vi "Create Schedule File (Main).vi"(0 "Team Info":T2, 5 "# of Fields":i32=1 min=1, 9 "Matches Per Team":i32=1 min=1, 11 "Back To Back Interval":i32 min=0) -> (4 "Match Array (indices)":i32[][](array[numeric]), 6 "# of Teams":i32, 8 "Team Info Out":T2, 10 "# of Quadrants":i32, 14 "Max H2H":i32, 15 "Total # of Matches":i32)   [LabVIEW 2013]
uses:
  Team Data Array.ctl
panel:
  in  "Tab Control":T1(tab)
  in  "Create schedule.csv":bool
  in  "Create By-Match CSV":bool
  in  "Cancel Button":bool
  in  "Create By-team CSV":bool
  out "error out":errorcluster
  in  "error in (no error)":errorcluster
  out "Progress":dbl(slide) scale=0.0..1.0
  in  "Output Folder":path
  in  "Entry Method":enum16{"Team Data Array", "Schedule Path"}(ring)
  in  "Team Info / Schedule File":path=path "Z:/Code/LabVIEW/[GEN2] FLL/schedule.csv"
  out "Flag Array":bool[][](array[boolean])
  out "H2H Flag":bool[][](array[boolean])
  out "H2H":i32[][](array[numeric])
  out "Match Array (numbers)":i32[][](array[numeric])
  out "By-Match Table":string[][](table)
  out "By-Team Table":string[][](table)
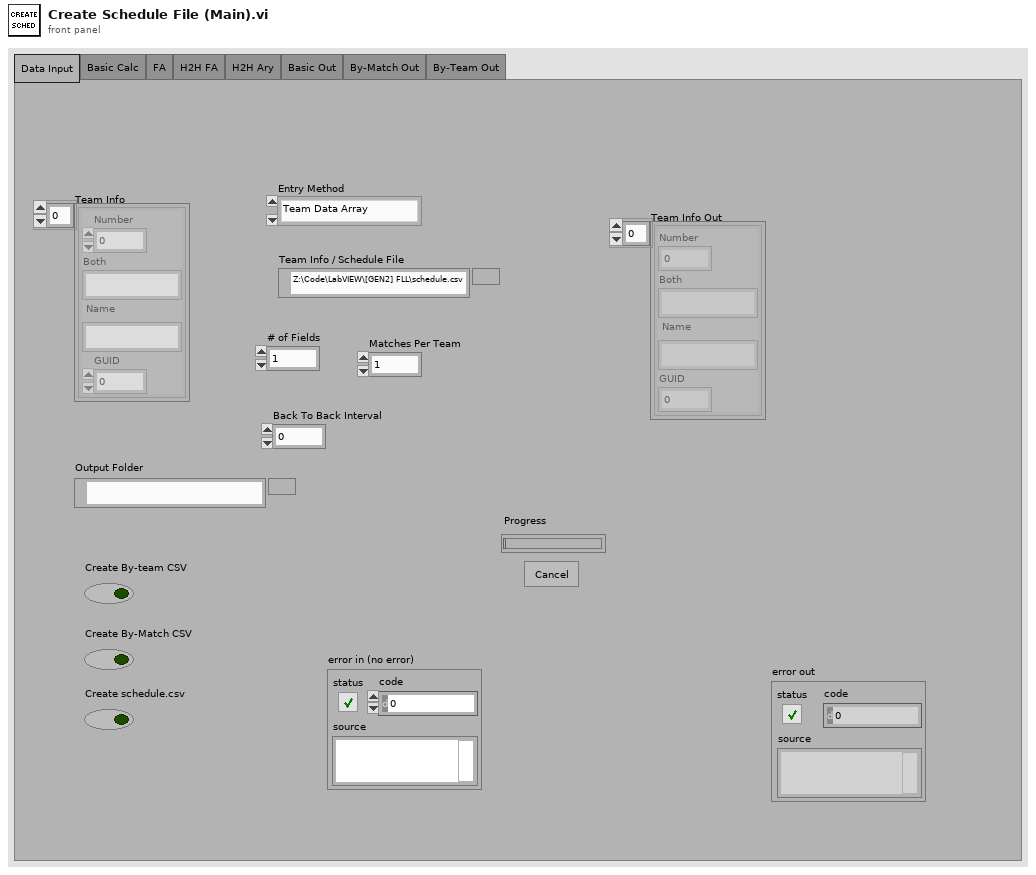
[diagram p1: front panel]
types:
  T1 = enum32{"Data Input", "Basic Calc", "FA", "H2H FA", "H2H Ary", "Basic Out", "By-Match Out", "By-Team Out"}
  T2 = typedef "Team Data Array.ctl" = cluster{"Number":u16, "Both":string, "Name":string, "GUID":u16}[]
  T3 = cluster{"Number":u16, "Both":string, "Name":string, "GUID":u16}
  T4 = cluster{"Total # of Matches":i32, "# of Fields":i32, "Matches Per Team":i32, "# of Teams":i32}
  T5 = cluster{"Row Headers":string[], "Column Headers":string[], "Items":string[][]}
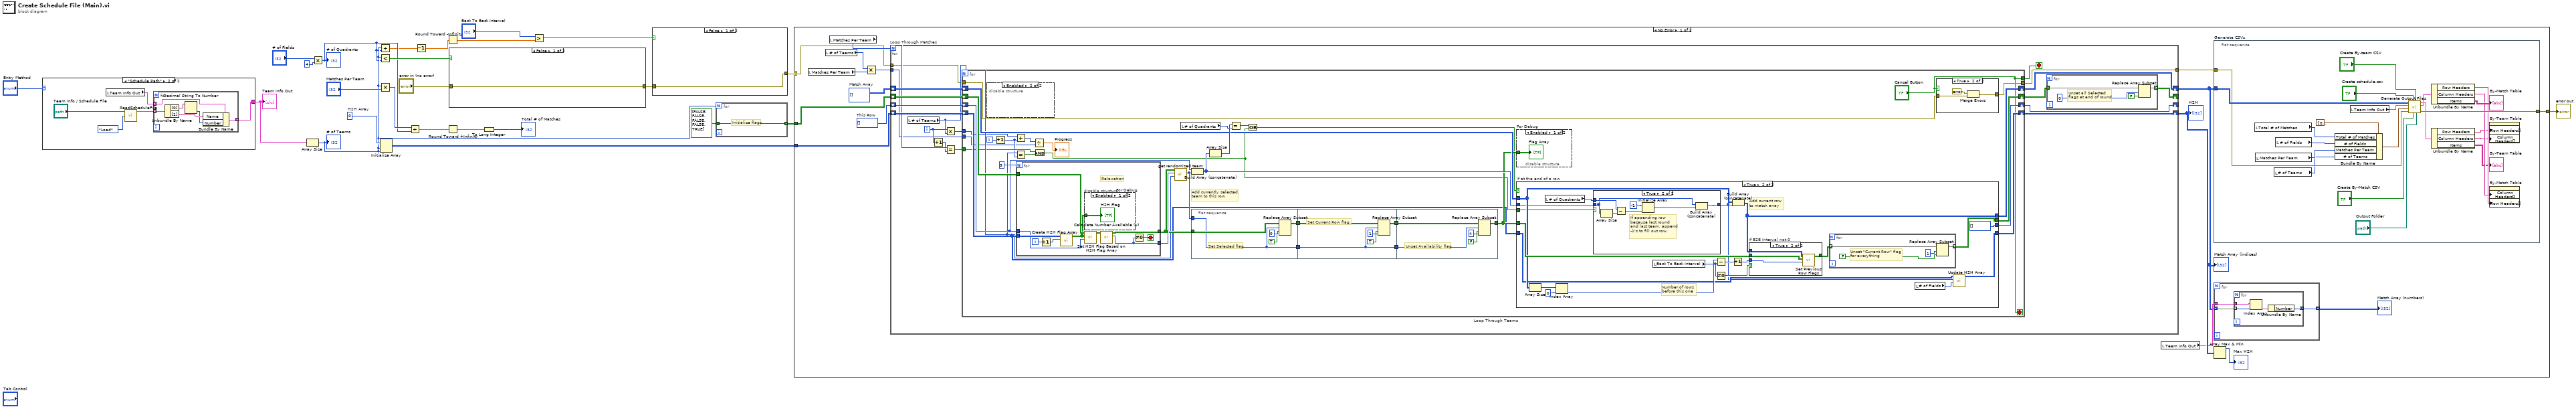
[diagram p0: block diagram]
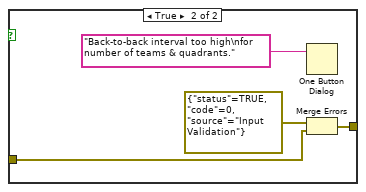
[diagram p2: hidden frame]
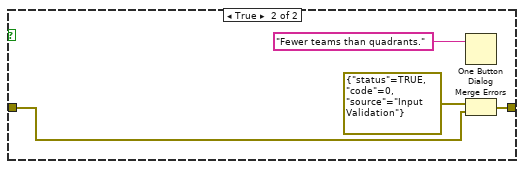
[diagram p3: hidden frame]
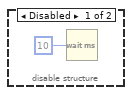
[diagram p7: hidden frame]
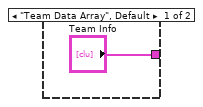
[diagram p12: hidden frame]
diagram:
  w17 = 0  # H2H Array
  n1 = case shown="\"Schedule Path\"" "Entry Method" {
    tunnel: ["Team Info" w28] -> w16
    frame "Team Data Array", Default {
    }
    frame "Schedule Path" {
      n2 = local read "Team Info Out"() -> (w27:T2)
      n3 = call "ReadScheduleFile.vi"("Enum"=enum16{"Load", "Get"}."Load", "Team Info / Schedule File"="Team Info / Schedule File") -> ("Team Information"=w30:cluster{string, "[0]":string, "[1]":string}[])  [unwired: 1 in, 5 out]
      n4 = for {
        tunnel: w30 -> [w36] mode=indexing
        tunnel: w27 -> [w37] mode=indexing
        tunnel: [w33] -> w28 mode=indexing
        n5 = Unbundle By Name(w36) -> ("[0]"=w34:string, "[1]"=w35:string)
        n6 = Decimal String To Number(string=w34) -> (number=w32:i32)  [unwired: 2 in, 1 out]
        n7 = Bundle By Name(cluster=w37, "Name"=w35, "Number"=w32) -> (w33:T3)
      }
    }
  }
  "Team Info Out" <- w16
  n8 = Array Size(array=w16) -> (size(s)=w9:i32)
  "# of Teams" <- w9
  n9 = Multiply(x="# of Fields", y=4) -> (x*y=w8:i32)
  "# of Quadrants" <- w8
  n10 = Divide(x=w9, y=w8) -> (x/y=w7:dbl)
  n11 = Less?(x=w9, y=w8) -> (x < y?=w11:bool)
  n12 = Multiply(x=w9, y="Matches Per Team") -> (x*y=w13:i32)
  n13 = Initialize Array(w17, w9, w9) -> (w24:i32[][])
  n14 = Divide(x=w13, y=w8) -> (x/y=w22:dbl)
  n15 = Decrement(x=w7) -> (x-1=w6:dbl)
  n16 = Round Toward -Infinity(1:w6) -> (0:w5:dbl)
  n17 = Round Toward +Infinity(x=w22) -> (ceil(x): smallest int >= x=w21:dbl)
  n18 = case shown="False" w11 {
    tunnel: "error in (no error)" -> [w38 w42]
    tunnel: [w38 w40] -> w10
    frame False {
    }
    frame True {
      n19 = One Button Dialog(message="Fewer teams than quadrants.") -> ()  [unwired: 1 in, 1 out]
      n20 = Merge Errors(errorcluster {"status"=TRUE, "code"=0, "source"="Input Validation"} ("error in"), w42) -> (w40:errorcluster)
    }
  }
  n21 = To Long Integer(number=w21) -> (32bit integer=→"Total # of Matches":i32)
  n22 = Greater?(x="Back To Back Interval", y=w5) -> (0:w3:bool)
  n23 = case shown="False" w3 {
    tunnel: w10 -> [w43 w47]
    tunnel: [w43 w45] -> w2
    frame False {
    }
    frame True {
      n24 = One Button Dialog(message="Back-to-back interval too high\nfor number of teams & quadrants.") -> ()  [unwired: 1 in, 1 out]
      n25 = Merge Errors(errorcluster {"status"=TRUE, "code"=0, "source"="Input Validation"} ("error in"), w47) -> (w45:errorcluster)
    }
  }
  n26 = for {
    N: w9 -> [_]
    tunnel: bool[] [FALSE, FALSE, FALSE, FALSE, TRUE] -> [w48]
    tunnel: [w48] -> w25 mode=indexing
    # "Initialize flags"
  }
  n27 = case shown="No Error" w2 {
    selector: w2 -> [w52 w225]
    tunnel: w25 -> [w64 _]
    tunnel: w24 -> [w63 _]
    tunnel: [w49 w225] -> w1
    frame No Error {
      w61 = i32[][] []  # Match Array
      w62 = i32[] []  # This Row
      n28 = local read "Matches Per Team"() -> (w54:i32)
      n29 = local read "# of Teams"() -> (w55:i32)
      n30 = local read "Matches Per Team"() -> (w56:i32)
      n31 = Multiply(x=w55, y=w54) -> (x*y=w53:i32)
      n32 = for "Loop Through Matches" {
        N: w56 -> [w103]
        shift-right: [w109] -> _
        shift-left: w62 -> [w110]
        shift-right: [w107] -> w51
        shift-left: w61 -> [w108]
        shift-right: [w106] -> w60
        shift-left: w63 -> [w112]
        shift-right: [w104] -> _
        shift-left: w64 -> [w111]
        tunnel: w53 -> [w97]
        tunnel: w52 -> [w95]
        tunnel: [w94] -> w50
        i -> [w99]
        stop <- w96 stop-if-true
        n33 = local read "# of Teams"() -> (w98:i32)
        n34 = Increment(x=w99) -> (x+1=w101:i32)
        n35 = Multiply(x=w99, y=w98) -> (x*y=w100:i32)
        n36 = Equal?(x=w103, y=w101) -> (x = y?=w102:bool)
        n37 = for "Loop Through Teams" {
          N: w98 -> [w132]
          shift-right: [w144] -> w105
          shift-left: w111 -> [w151]
          shift-right: [w148] -> w109
          shift-left: w110 -> [w134]
          shift-right: [w146] -> w107
          shift-left: w108 -> [w147]
          shift-right: [w145] -> w106
          shift-left: w112 -> [w135]
          tunnel: w102 -> [w130]
          tunnel: w100 -> [w126]
          tunnel: w97 -> [w121]
          tunnel: ["Cancel Button"] -> w96
          tunnel: w95 -> [w118]
          tunnel: [w117] -> w94
          i -> [w133]
          stop <- "Cancel Button" stop-if-true
          # "Add currently selected\nteam to this row"
          n38 = disable-structure shown="Enabled" {
            frame Disabled {
              n39 = Wait (ms)(milliseconds to wait=u32 10) -> ()  [unwired: 1 out]
            }
            frame Enabled {
            }
          }
          n40 = Increment(x=w133) -> (x+1=w125:i32)
          n41 = Add(x=w126, y=w125) -> (x+y=w124:i32)
          n42 = Equal?(x=w132, y=w125) -> (x = y?=w131:bool)
          n43 = for {
            N: 9 -> [_]
            tunnel: w151 -> [w159]
            tunnel: [w162] -> w141
            tunnel: [w165] -> w143
            tunnel: w135 -> [w163]
            tunnel: w134 -> [w157]
            i -> [w164]
            stop <- w156 stop-if-true
            # "Relaxation"
            n44 = Increment(x=w164) -> (x+1=w161:i32)
            n45 = call "Create H2H Flag Array.vi"("H2H Cutoff"=w161, "H2H Array"=w163) -> ("H2H Flag"=w158:bool[][])  [unwired: 9 in]
            n46 = disable-structure "For Debug" shown="Enabled" {
              disable-tunnel: w158 -> [w166 _]
              frame Enabled {
                "H2H Flag" <- w166
              }
              frame Disabled {
              }
            }
            n47 = call "Set H2H Flag Based on H2H Flag Array.vi"("This Row"=w157, "H2H Flag Array"=w158, "Flag Array"=w159) -> ("Flag Array Out"=w160:bool[][])  [unwired: 8 in]
            n48 = call "Calculate Number Available (u).vi"("Flag Array"=w160) -> ("u"=w165:i32, "Flag Array Out"=w162:bool[][])  [unwired: 9 in]
            n49 = Not Equal To 0?(x=w165) -> (x != 0?=w156:bool)
          }
          n50 = Divide(x=w124, y=w121) -> (x/y=→"Progress":dbl)
          n51 = And(x=w130, y=w131) -> (x .and. y?=w127:bool)
          n52 = call "get randomized team.vi"("# of Teams"=w132, "u"=w143, "Flag Array"=w141) -> ("This Team"=w142:i32)  [unwired: 8 in]
          n53 = local read "# of Quadrants"() -> (w122:i32)
          n54 = Build Array (concatenate)(w134, w142) -> (w149:i32[])
          n55 = flat-sequence {
            tunnel: w142 -> [w169]
            tunnel: w141 -> [w170]
            tunnel: [w171] -> w140
            tunnel: [w169] -> w139
            tunnel: w140 -> [w176]
            tunnel: w139 -> [w174]
            tunnel: [w175] -> w138
            tunnel: [w174] -> w136
            tunnel: [w180] -> w137
            tunnel: w138 -> [w181]
            tunnel: w136 -> [w179]
            frame #0 {
              # "Set Selected flag"
              n56 = Replace Array Subset(array=w170, new element=TRUE ("new element/subarray"), index (row)=w169, index (col)=0 ("disabled index (col)")) -> (w171:bool[][])
            }
            frame #1 {
              # "Set Current Row flag."
              n57 = Replace Array Subset(array=w176, new element=TRUE ("new element/subarray"), index (row)=w174, index (col)=1 ("disabled index (col)")) -> (w175:bool[][])
            }
            frame #2 {
              # "Unset Availability flag"
              n58 = Replace Array Subset(array=w181, new element=FALSE ("new element/subarray"), index (row)=w179, index (col)=4 ("disabled index (col)")) -> (w180:bool[][])
            }
          }
          n59 = Array Size(array=w149) -> (size(s)=w150:i32)
          n60 = Equal?(x=w150, y=w122) -> (x = y?=w129:bool)
          n61 = Or(x=w129, y=w127) -> (x .or. y?=w128:bool)
          n62 = disable-structure "For Debug" shown="Enabled" {
            disable-tunnel: w137 -> [w167 _]
            frame Enabled {
              "Flag Array" <- w167
            }
            frame Disabled {
            }
          }
          n63 = case "If at the end of a row" shown="True" w128 {
            tunnel: w149 -> [w187 w193]
            tunnel: [w187 i32[] []] -> w148
            tunnel: w147 -> [w186 w205]
            tunnel: [w186 w201] -> w146
            tunnel: w135 -> [w185 w195]
            tunnel: [w185 w194] -> w145
            tunnel: w137 -> [w184 w206]
            tunnel: [w184 w197] -> w144
            tunnel: w127 -> [_ w191]
            frame False {
            }
            frame True {
              # "Number of rows\nbefore this one"
              # "Add current row\nto match array"
              n64 = Array Size(array=w205) -> (size(s)=w204:i32[])
              n65 = local read "# of Quadrants"() -> (w188:i32)
              n66 = Index Array(array=w204, index=0) -> (element=w202:i32)
              n67 = case shown="True" w191 {
                tunnel: w193 -> [w208 w210]
                tunnel: [w208 w211] -> w192
                tunnel: w188 -> [_ w215]
                frame False {
                }
                frame True {
                  # "If appending row\nbecause last round \nand last team, append\n-1's to fill out row."
                  n68 = Array Size(array=w210) -> (size(s)=w214:i32)
                  n69 = Subtract(x=w215, y=w214) -> (x-y=w213:i32)
                  n70 = Initialize Array(-1, w213) -> (w209:i32[])
                  n71 = Build Array (concatenate)(w210, w209) -> (w211:i32[])
                }
              }
              n72 = local read "Back To Back Interval"() -> (w190:i32)
              n73 = Subtract(x=w202, y=w190) -> (x-y=w200:i32)
              n74 = Not Equal To 0?(x=w190) -> (x != 0?=w196:bool)
              n75 = Increment(x=w200) -> (x+1=w199:i32)
              n76 = Build Array (concatenate)(w205, w192) -> (w201:i32[][])
              n77 = case "If B2B Interval not 0" shown="True" w196 {
                tunnel: w206 -> [w216 w219]
                tunnel: w201 -> [_ w220]
                tunnel: w199 -> [_ w218]
                tunnel: [w216 w217] -> w198
                frame False {
                }
                frame True {
                  n78 = call "Set Previous Row Flags.vi"("Cutoff"=w218, "Flag Array"=w219, "Match Array"=w220) -> ("Flag Array Out"=w217:bool[][])  [unwired: 8 in]
                }
              }
              n79 = for {
                tunnel: w198 -> [w224] mode=indexing
                tunnel: [w221] -> w197 mode=indexing
                # "Unset \"Current Row\" flag\nfor everything"
                n80 = Replace Array Subset(array=w224, new element=FALSE ("new element/subarray"), index=1) -> (w221:bool[])
              }
              n81 = local read "# of Fields"() -> (w189:i32)
              n82 = call "Update H2H Array.vi"("# of Fields"=w189, "New Row"=w192, "H2H Array"=w195) -> ("H2H Array Out"=w194:i32[][])  [unwired: 8 in]
            }
          }
          n83 = case shown="True" "Cancel Button" {
            tunnel: w118 -> [w152 w155]
            tunnel: [w152 w153] -> w117
            frame False {
            }
            frame True {
              n84 = Merge Errors(errorcluster {"status"=TRUE, "code"=0, "source"="Cancelled"} ("error in"), w155) -> (w153:errorcluster)
            }
          }
        }
        n85 = for {
          tunnel: w105 -> [w115] mode=indexing
          tunnel: [w114] -> w104 mode=indexing
          # "Unset all Selected\nflags at end of round"
          n86 = Replace Array Subset(array=w115, new element=FALSE ("new element/subarray"), index=0) -> (w114:bool[])
        }
      }
      "Match Array (indices)" <- w51
      "H2H" <- w60
      n87 = local read "Team Info Out"() -> (w58:T2)
      n88 = flat-sequence "Generate CSVs" {
        tunnel: w51 -> [w86]
        tunnel: w50 -> [w81]
        tunnel: [w80] -> w49
        frame #0 {
          n89 = local read "Total # of Matches"() -> (w76:i32)
          n90 = local read "Matches Per Team"() -> (w74:i32)
          n91 = local read "# of Teams"() -> (w73:i32)
          n92 = local read "# of Fields"() -> (w75:i32)
          n93 = Bundle By Name(cluster=T4 {"Total # of Matches"=0, "# of Fields"=0, "Matches Per Team"=0, "# of Teams"=0} ("General Data"), "Total # of Matches"=w76, "# of Fields"=w75, "Matches Per Team"=w74, "# of Teams"=w73) -> (w77:T4)
          n94 = local read "Team Info Out"() -> (w79:T2)
          n95 = call "Generate Output Files.vi"("Output Folder"="Output Folder", "Create By-Team CSV"="Create By-team CSV", "Create By-Match CSV"="Create By-Match CSV", "Create schedule.csv"="Create schedule.csv", "error in (no error)"=w81, "General Data"=w77, "Team Info"=w79, "Match Array"=w86) -> ("error out"=w80:errorcluster, "By Match List"=w72:T5, "By Team List"=w68:T5)  [unwired: 1 in]
          n96 = Unbundle By Name(w72) -> ("Row Headers"=w69:string[], "Column Headers"=w70:string[], "Items"=→"By-Match Table":string[][])
          n97 = Unbundle By Name(w68) -> ("Row Headers"=w66:string[], "Column Headers"=w65:string[], "Items"=→"By-Team Table":string[][])
          n98 = property on="By-Team Table" class="Tbl (strict)"("Row Headers[]"=w66, "Column Headers[]"=w65) -> ()  [unwired: 2 in, 2 out]
          n99 = property on="By-Match Table" class="Tbl (strict)"("Column Headers[]"=w70, "Row Headers[]"=w69) -> ()  [unwired: 2 in, 2 out]
        }
      }
      n100 = for {
        tunnel: w51 -> [w89] mode=indexing
        tunnel: w58 -> [w88]
        tunnel: [w87] -> w57 mode=indexing
        n101 = for {
          tunnel: w89 -> [w92] mode=indexing
          tunnel: w88 -> [w93]
          tunnel: [w90] -> w87 mode=indexing
          n102 = Index Array(array=w93, index=w92) -> (element=w91:T3)
          n103 = Unbundle By Name(w91) -> ("Number"=w90:u16)
        }
      }
      "Match Array (numbers)" <- w57
      n104 = Array Max & Min(array=w60) -> (max value=→"Max H2H":i32)  [unwired: 3 out]
    }
    frame Error {
    }
  }
  "error out" <- w1
